vi "EVM_Sweep_Only.vi"() -> ()   [LabVIEW 2023, in "EVM.lvlib"]
uses:
  EVM.lvlib
  lib/Keysight/Keysight.lvlib
panel:
  in  "Type":enum16{"Default", "E6680A"}(ring)=enum."E6680A"
  in  "Waiting Time(ms)":u32=1000
  in  "FileNote":string
  out "SG Power":i32
  in  "Stop Power":i32=8
  in  "Start Power":i32=-40
  in  "SG":refnum<visa-resource-name>="TCPIP0::192.168.100.200::inst0::INSTR"
  in  "AvgTimes":i32=5
  in  "SA":refnum<visa-resource-name>="TCPIP0::192.168.100.230::inst0::INSTR"
  out "Spectrum Data":cluster{"X":dbl, "Y":dbl}[](graph)
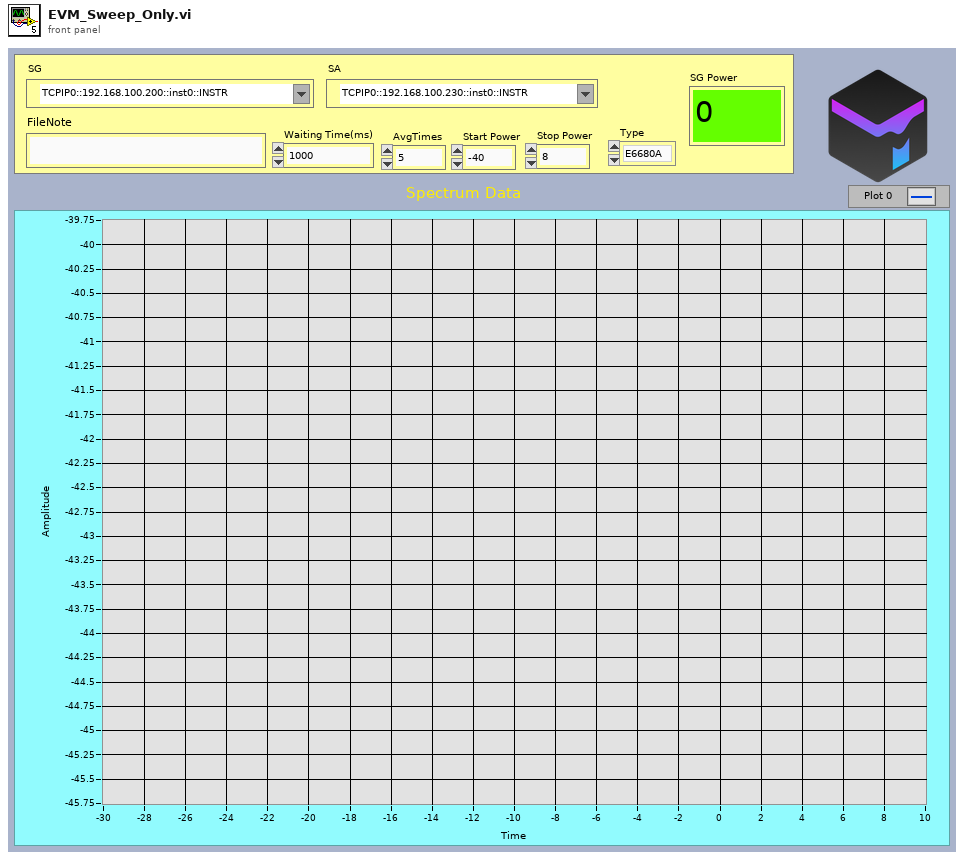
[diagram p1: front panel]
types:
  T1 = cluster{"RMS EVM Avg (dB)":dbl, "RMS EVM Avg (%)":dbl, "Frequency Error Avg (Hz)":dbl, "Avg Burst Power Avg (dBm)":dbl, "Frequency Error Avg (ppm)":dbl}
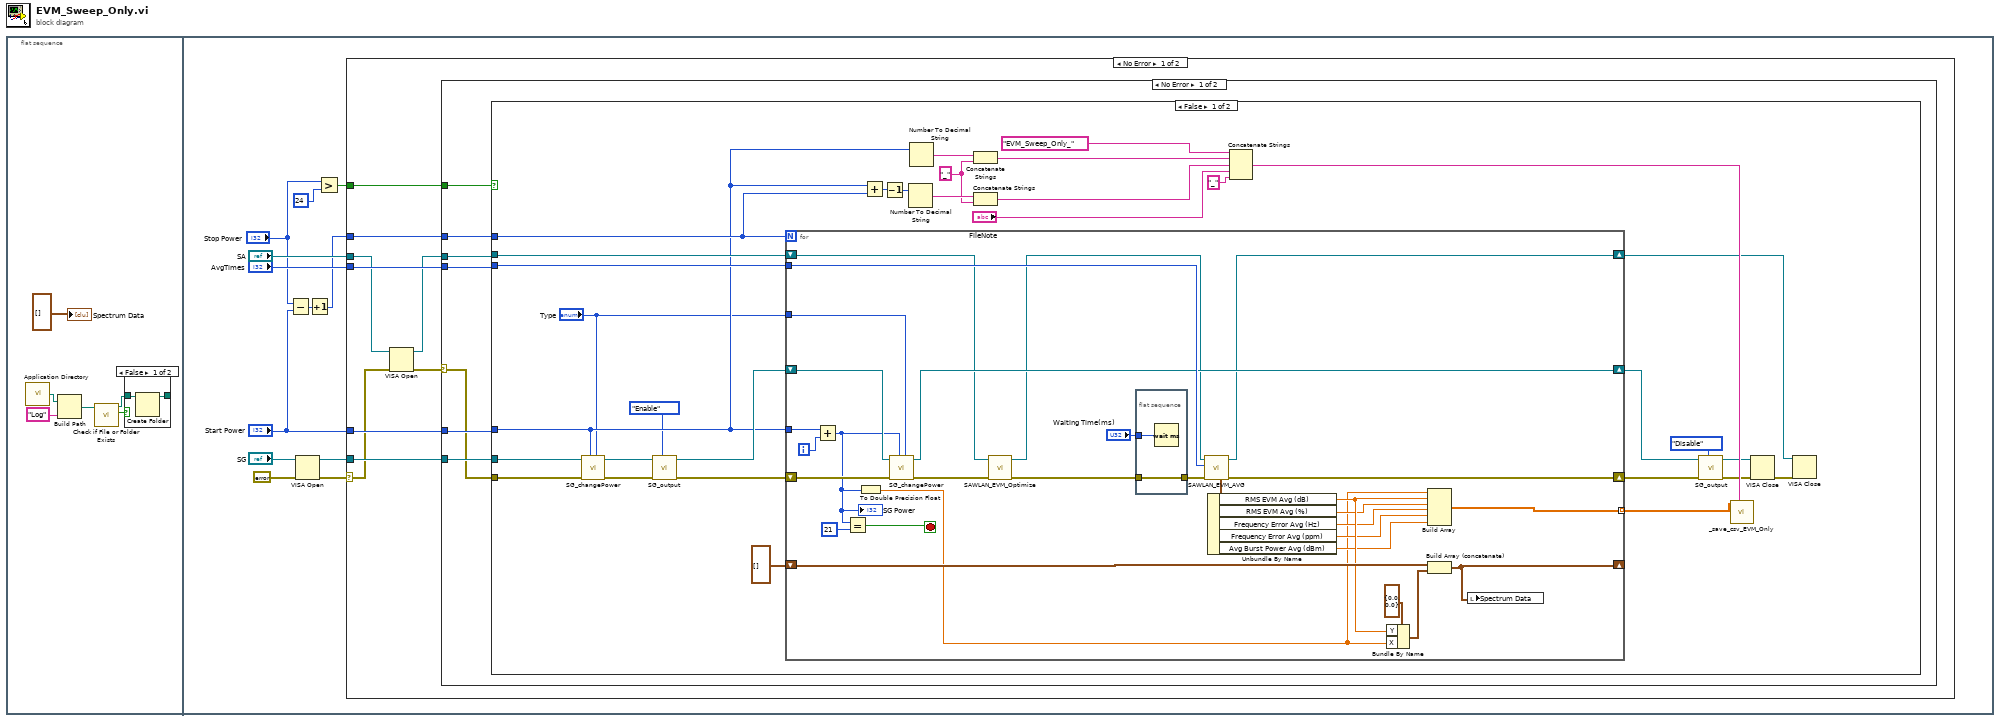
[diagram p0: block diagram]
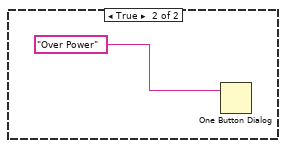
[diagram p3: hidden frame]
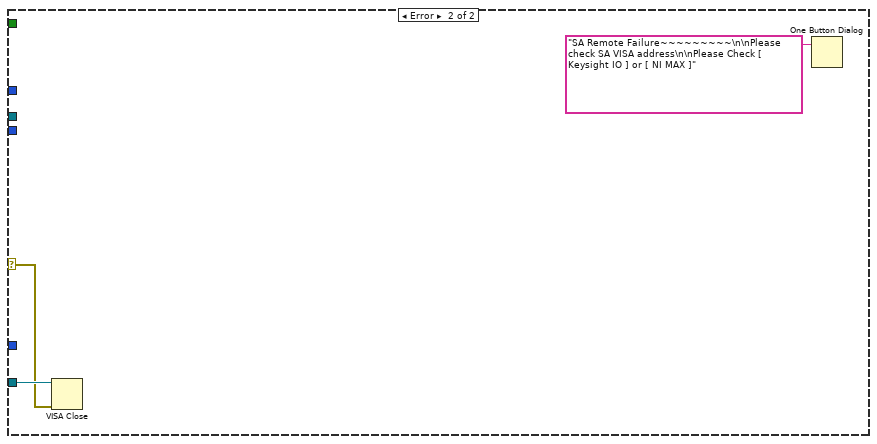
[diagram p4: hidden frame]
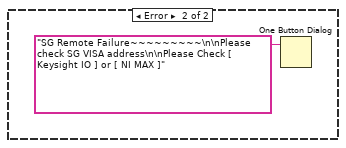
[diagram p5: hidden frame]
diagram:
  n1 = flat-sequence {
    frame #0 {
      n2 = call <vilib>:"Application Directory.vi"() -> ("Application Directory"=w5:path)
      n3 = Build Path(base path=w5, name or relative path="Log") -> (appended path=w2:path)
      n4 = call <vilib>:"Check if File or Folder Exists.vi"("path"=w2) -> ("file or folder exists?"=w4:bool, "dup path"=w3:path)  [unwired: 8 in, 1 out]
      n5 = case shown="False" w4 {
        tunnel: w3 -> [w8 w9]
        tunnel: [w7 w9] -> _
        frame False {
          n6 = Create Folder(path (use dialog)=w8) -> (created path=w7:path)  [unwired: 2 in, 2 out]
        }
        frame True {
        }
      }
      "Spectrum Data" <- cluster{"X":dbl, "Y":dbl}[] [] ("XY Graph")
    }
    frame #1 {
      n7 = Subtract(x="Stop Power", y="Start Power") -> (x-y=w17:i32)
      n8 = VISA Open(error in (no error)=errorcluster {"status"=FALSE, "code"=0, "source"=""}, VISA resource name="SG") -> (VISA resource name=w11:refnum<visa-resource-name>, error out=w10:errorcluster)  [unwired: 3 in]
      n9 = Increment(x=w17) -> (x+1=w16:i32)
      n10 = Greater?(x="Stop Power", y=24) -> (0:w20:bool)
      n11 = case shown="No Error" w10 {
        selector: w10 -> [w25 _]
        tunnel: "SA" -> [w23 _]
        tunnel: w20 -> [w30 _]
        tunnel: "Start Power" -> [w29 _]
        tunnel: "AvgTimes" -> [w28 _]
        tunnel: w16 -> [w27 _]
        tunnel: w11 -> [w26 _]
        frame No Error {
          n12 = VISA Open(error in (no error)=w25, VISA resource name=w23) -> (VISA resource name=w22:refnum<visa-resource-name>, error out=w24:errorcluster)  [unwired: 3 in]
          n13 = case shown="No Error" w24 {
            selector: w24 -> [w31 w103]
            tunnel: w22 -> [w37 _]
            tunnel: w30 -> [w36 _]
            tunnel: w29 -> [w35 _]
            tunnel: w28 -> [w34 _]
            tunnel: w27 -> [w33 _]
            tunnel: w26 -> [w32 w104]
            frame No Error {
              n14 = case shown="False" w36 {
                tunnel: w37 -> [w69 _]
                tunnel: w34 -> [w68 _]
                tunnel: w35 -> [w42 _]
                tunnel: w31 -> [w55 _]
                tunnel: w32 -> [w54 _]
                tunnel: w33 -> [w52 _]
                frame False {
                  w61 = "_"
                  n15 = call "SG_changePower.vi"("Type"="Type", "dBm"=w42, "error in"=w55, "VISA in"=w54) -> ("error out"=w56:errorcluster, "VISA out"=w53:refnum<visa-resource-name>)  [unwired: 5 in, 1 out]
                  n16 = call "SG_output.vi"("Func."=enum16{"Disable", "Enable"}."Enable", "error in"=w56, "VISA in"=w53) -> ("error out"=w67:errorcluster, "VISA out"=w51:refnum<visa-resource-name>)  [unwired: 7 in]
                  n17 = for {
                    N: w52 -> [_]
                    tunnel: w68 -> [w99]
                    tunnel: w42 -> [w96]
                    shift-right: [w91] -> w66
                    shift-left: w67 -> [w98]
                    shift-right: [w93] -> w50
                    shift-left: w51 -> [w92]
                    shift-right: [w88] -> w43
                    shift-left: w69 -> [w80]
                    shift-right: [w84] -> _
                    shift-left: cluster{"X":dbl, "Y":dbl}[] [] ("XY Graph") -> [w86]
                    tunnel: [w72] -> w40 mode=indexing
                    tunnel: "Type" -> [w70]
                    i -> [w97]
                    stop <- w94 stop-if-true
                    n18 = Add(x=w96, y=w97) -> (x+y=w83:i32)
                    "SG Power" <- w83
                    n19 = Equal?(x=w83, y=21) -> (x = y?=w94:bool)
                    n20 = To Double Precision Float(number=w83) -> (double precision float=w71:dbl)
                    n21 = call "SG_changePower.vi"("Type"=w70, "dBm"=w83, "error in"=w98, "VISA in"=w92) -> ("error out"=w82:errorcluster, "VISA out"=w93:refnum<visa-resource-name>)  [unwired: 5 in, 1 out]
                    n22 = call "SAWLAN_EVM_Optimize.vi"("error in"=w82, "VISA in"=w80) -> ("error out"=w81:errorcluster, "VISA out"=w79:refnum<visa-resource-name>)  [unwired: 8 in]
                    n23 = flat-sequence {
                      tunnel: w81 -> [w101]
                      tunnel: [w101] -> w90
                      tunnel: "Waiting Time(ms)" -> [w100]
                      frame #0 {
                        n24 = Wait (ms)(milliseconds to wait=w100) -> ()  [unwired: 1 out]
                      }
                    }
                    n25 = call "SAWLAN_EVM_AVG.vi"("error in (no error)"=w90, "AvgTimes"=w99, "VISA resource name"=w79) -> ("error out"=w91:errorcluster, "VISA resource name out"=w88:refnum<visa-resource-name>, "output"=w78:T1)  [unwired: 6 in]
                    n26 = Unbundle By Name(w78) -> ("RMS EVM Avg (dB)"=w77:dbl, "RMS EVM Avg (%)"=w76:dbl, "Frequency Error Avg (Hz)"=w75:dbl, "Frequency Error Avg (ppm)"=w74:dbl, "Avg Burst Power Avg (dBm)"=w73:dbl)
                    n27 = Bundle By Name(cluster=cluster{"X":dbl, "Y":dbl} {"X"=0.0, "Y"=0.0} ("element"), "Y"=w77, "X"=w71) -> (w85:cluster{"X":dbl, "Y":dbl})
                    n28 = Build Array(w71, w77, w76, w75, w74, w73) -> (w72:dbl[])
                    n29 = Build Array (concatenate)(w86, w85) -> (w84:cluster{"X":dbl, "Y":dbl}[])
                    n30 = local write "Spectrum Data"(w84) -> ()
                  }
                  n31 = Add(x=w42, y=w52) -> (x+y=w65:i32)
                  n32 = Decrement(x=w65) -> (x-1=w64:i32)
                  n33 = Number To Decimal String(number=w64) -> (decimal integer string=w62:string)  [unwired: 1 in]
                  n34 = Number To Decimal String(number=w42) -> (decimal integer string=w63:string)  [unwired: 1 in]
                  n35 = Concatenate Strings(w63, w61) -> (w59:string)
                  n36 = Concatenate Strings(w62, w61) -> (w58:string)
                  n37 = Concatenate Strings("EVM_Sweep_Only_" ("delimiter (\\t)"), w59, w58, "FileNote", "_") -> (w57:string)
                  n38 = call "SG_output.vi"("Func."=enum16{"Disable", "Enable"}."Disable", "error in"=w66, "VISA in"=w50) -> ("error out"=w46:errorcluster, "VISA out"=w45:refnum<visa-resource-name>)  [unwired: 7 in]
                  n39 = call "_save_csv_EVM_Only.vi"("delimiter (\\t)"=w57, "Data"=w40) -> ()  [unwired: 9 in, 1 out]
                  n40 = VISA Close(VISA resource name=w45, error in (no error)=w46) -> (error out=w44:errorcluster)
                  n41 = VISA Close(VISA resource name=w43, error in (no error)=w44) -> ()  [unwired: 1 out]
                }
                frame True {
                  n42 = One Button Dialog(message="Over Power") -> ()  [unwired: 1 in, 1 out]
                }
              }
            }
            frame Error {
              n43 = VISA Close(VISA resource name=w104, error in (no error)=w103) -> ()  [unwired: 1 out]
              n44 = One Button Dialog(message="SA Remote Failure~~~~~~~~~\n\nPlease check SA VISA address\n\nPlease Check [ Keysight IO ] or [ NI MAX ]") -> ()  [unwired: 1 in, 1 out]
            }
          }
        }
        frame Error {
          n45 = One Button Dialog(message="SG Remote Failure~~~~~~~~~\n\nPlease check SG VISA address\n\nPlease Check [ Keysight IO ] or [ NI MAX ]") -> ()  [unwired: 1 in, 1 out]
        }
      }
    }
  }
